vi "Get Supported Targets.vi"(8 "error in":errorcluster, 11 "Asynchronous Component Configuration In":refnum<class "asynchronous execution module configuration.lvclass">) -> (0 "error out":errorcluster, 2 "supported targets":T1[](array[typedef]), 3 "Asynchronous Component Configuration Out":refnum<class "asynchronous execution module configuration.lvclass">)   [LabVIEW 2013, in "asynchronous execution module configuration.lvclass"]
doc: "Provides an interface for determining the targets supported by a given component configuration/runtime class pairing. This should be overridden by any useful child class."
uses:
  asynchronous execution module configuration.lvclass
  <vilib>/NI/Tag Bus Module Framework/root configuration/Target Types.ctl
  asynchronous execution module configuration.lvclass/asynchronous execution module configuration.ctl
  <vilib>/NI/Tag Bus Module Framework/module configuration/TBM module configuration.lvclass
  <vilib>/NI/Tag Bus Module Framework/root configuration/TBM configuration.lvclass
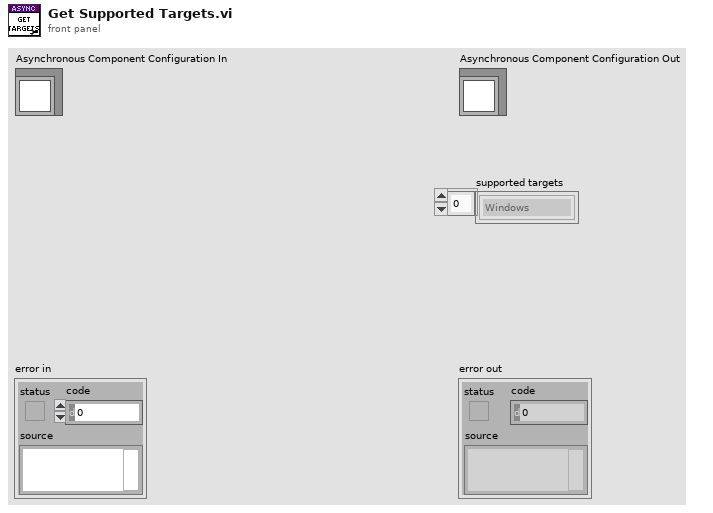
[diagram p1: front panel]
types:
  T1 = typedef "TBM configuration.lvclass/Target Types.ctl" = enum16{"Windows", "Mac", "Linux", "Linux RT ARM", "VxWorks", "Pharlap", "Other", "Linux RT x64"}
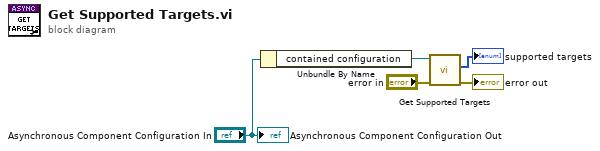
[diagram p0: block diagram]
diagram:
  n1 = Unbundle By Name("Asynchronous Component Configuration In") -> ("contained configuration"=w4:refnum<class "TBM module configuration.lvclass">)
  n2 = call-dynamic "Get Supported Targets.vi"("error in"="error in", "module configuration in"=w4) -> ("error out"=→"error out":errorcluster, "supported targets"=→"supported targets":T1[])  [unwired: 7 in, 1 out]
  "Asynchronous Component Configuration Out" <- "Asynchronous Component Configuration In"
